vi "获取触发信号.vi"(9 "截取信号长度":i32=256, 10 "触发":dbl, 11 "输入信号":dbl[](array[numeric])) -> (1 "触发":bool, 3 "截取信号":dbl[](array[numeric]))   [LabVIEW 2016]
uses:
  <vilib>/Analysis/NI_AALPro.lvlib
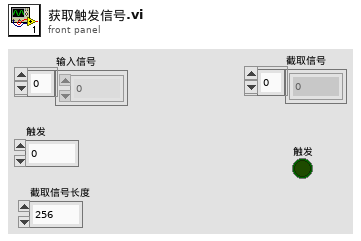
[diagram p1: front panel]
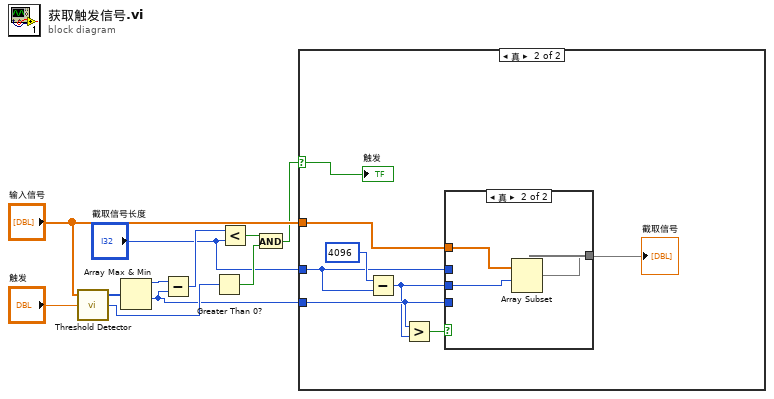
[diagram p0: block diagram]
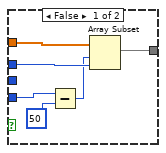
[diagram p3: hidden frame]
diagram:
  n1 = call <vilib>:"Threshold Detector.vi"("threshold"="触发", "X"="输入信号") -> ("count"=w9:i32, "Indices"=w8:i32[])  [unwired: 1 in, 1 out]
  n2 = Array Max & Min(array=w8) -> (max value=w7:i32, min value=w1:i32)  [unwired: 2 out]
  n3 = Subtract(x=w7, y=w1) -> (x-y=w6:i32)
  n4 = Greater Than 0?(x=w9) -> (x > 0?=w4:bool)
  n5 = Less?(x=w6, y="截取信号长度") -> (x < y?=w5:bool)
  n6 = And(x=w5, y=w4) -> (x .and. y?=w3:bool)
  n7 = case shown="真" w3 {
    selector: w3 -> [_ w19]
    tunnel: "输入信号" -> [_ w18]
    tunnel: "截取信号长度" -> [_ w15]
    tunnel: w1 -> [_ w14]
    frame False {
    }
    frame True {
      n8 = Subtract(x=4096, y=w15) -> (x-y=w12:i32)
      n9 = Greater?(x=w14, y=w12) -> (0:w13:bool)
      n10 = case shown="真" w13 {
        tunnel: w18 -> [w25 w27]
        tunnel: [w24 w28] -> w17
        tunnel: w15 -> [w23 _]
        tunnel: w14 -> [w21 _]
        tunnel: w12 -> [_ w26]
        frame False {
          n11 = Subtract(x=w21, y=50) -> (x-y=w22:i32)
          n12 = Array Subset(array=w25, index=w22, length=w23) -> (w24:dbl[])
        }
        frame True {
          n13 = Array Subset(array=w27, index=w26) -> (w28:dbl[])  [unwired: 1 in]
        }
      }
      "截取信号" <- w17
      "触发" <- w19
    }
  }
